vi "FieldDisp_Element_Disp.vi"(6 "Visible":bool=TRUE, 9 "Element Pose":T2 {"ROTATION"."SIN" format="%13.4f"; "ROTATION"."COS" format="%13.4f"; "ROTATION"."VALUE" format="%13.4f"; "TRANSLATION"."Y" format="%14.3f"; "TRANSLATION"."X" format="%14.3f"}, 11 "Element Info":T1) -> ()   [LabVIEW 2019, in "Trajectory_Library.lvlib"]
doc: "Displays, moves and rotates the field element on the display. \n\nInputs:\n - Element Info -- cluster -- information defining the field element.\n - Element Pose -- Pose2d -- Location and orientation of the field element.\n\nOutputs:\n -- NONE --"
uses:
  Trajectory_Library.lvlib
  TypeDef/POSE2D.ctl
  TypeDef/TRANSLATION2D.ctl
  TypeDef/ROTATION2D.ctl
  TypeDef/FieldDisp_FieldElement.ctl
  <vilib>/picture/pixmap.llb/Flatten Pixmap.vi
  <vilib>/picture/pictutil.llb/Create Mask.vi
  <vilib>/picture/picture.llb/Draw Flattened Pixmap.vi
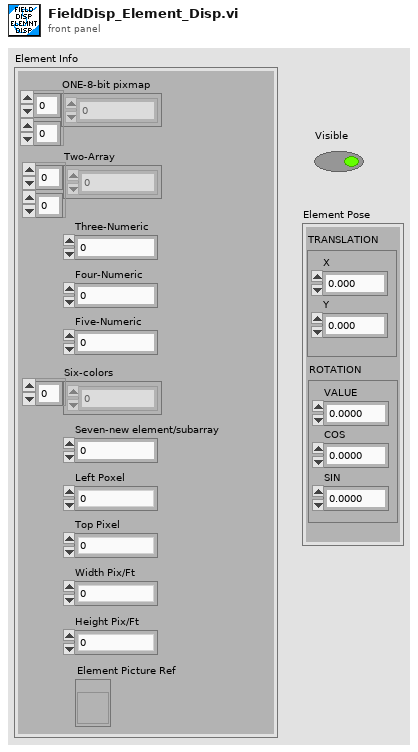
[diagram p1: front panel]
types:
  T1 = typedef "Trajectory_Library.lvlib/FieldDisp_FieldElement.ctl" = cluster{"ONE-8-bit pixmap":u8[][], "Two-Array":cdb[][], "Three-Numeric":i32, "Four-Numeric":i32, "Five-Numeric":cdb, "Six-colors":u32[], "Seven-new element/subarray":u32, "Left Poxel":dbl, "Top Pixel":dbl, "Width Pix/Ft":dbl, "Height Pix/Ft":dbl, "Element Picture Ref":refnum<vi>}
  T2 = typedef "Trajectory_Library.lvlib/POSE2D.ctl" = cluster{"TRANSLATION":T3, "ROTATION":T4}
  T3 = typedef "Trajectory_Library.lvlib/TRANSLATION2D.ctl" = cluster{"X":dbl, "Y":dbl}
  T4 = typedef "Trajectory_Library.lvlib/ROTATION2D.ctl" = cluster{"VALUE":dbl, "COS":dbl, "SIN":dbl}
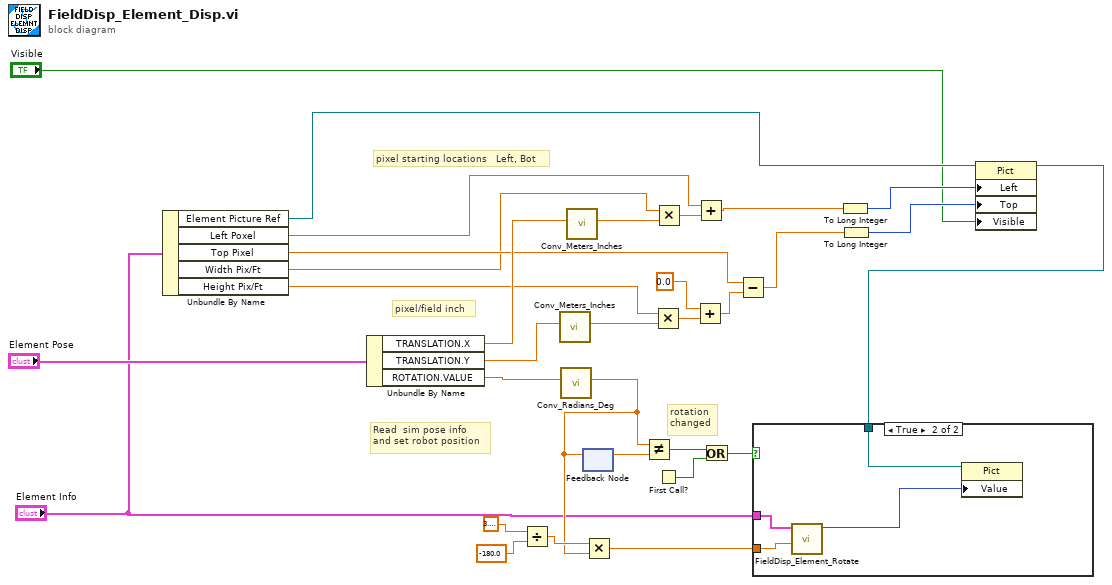
[diagram p0: block diagram]
diagram:
  # "pixel starting locations   Left, Bot"
  # "Read  sim pose info \nand set robot position"
  # "pixel/field inch"
  # "rotation\nchanged"
  n1 = Unbundle By Name("Element Info") -> ("Element Picture Ref"=w2:refnum<vi>, "Left Poxel"=w6:dbl, "Top Pixel"=w5:dbl, "Width Pix/Ft"=w4:dbl, "Height Pix/Ft"=w3:dbl)
  n2 = Unbundle By Name("Element Pose") -> ("TRANSLATION.X"=w15:dbl, "TRANSLATION.Y"=w16:dbl, "ROTATION.VALUE"=w18:dbl)
  n3 = Divide(x=3.141592653589793, y=-180.0 ("value")) -> (x/y=w27:dbl)
  n4 = call "Conv_Meters_Inches.vi"("Meters"=w16) -> ("Inches"=w22:dbl)  [unwired: 10 in]
  n5 = call "Conv_Radians_Deg.vi"("Radians"=w18) -> ("Degrees"=w17:dbl)  [unwired: 10 in]
  n6 = call "Conv_Meters_Inches.vi"("Meters"=w15) -> ("Inches"=w23:dbl)  [unwired: 10 in]
  n7 = feedback #1() -> (w8:dbl)  [unwired: 1 in]
  n8 = feedback-in #1(w17) -> ()
  n9 = Multiply(x=w27, y=w17) -> (x*y=w19:dbl)
  n10 = Not Equal?(x=w17, y=w8) -> (x != y?=w14:bool)
  n11 = Multiply(x=w3, y=w22) -> (x*y=w10:dbl)
  n12 = Multiply(x=w4, y=w23) -> (x*y=w9:dbl)
  n13 = First Call?() -> (First Call?: T/F=w28:bool)
  n14 = Add(x=0.0, y=w10) -> (x+y=w12:dbl)
  n15 = Add(x=w6, y=w9) -> (x+y=w20:dbl)
  n16 = Or(x=w14, y=w28) -> (x .or. y?=w13:bool)
  n17 = Subtract(x=w5, y=w12) -> (x-y=w21:dbl)
  n18 = To Long Integer(number=w20) -> (32bit integer=w29:i32)
  n19 = To Long Integer(number=w21) -> (32bit integer=w30:i32)
  n20 = property class="Pict"(reference=w2, "Left"=w29, "Top"=w30, "Visible"="Visible") -> (reference out=w31:refnum<vi>)  [unwired: 1 in, 1 out]
  n21 = case shown="True" w13 {
    tunnel: w19 -> [_ w34]
    tunnel: "Element Info" -> [_ w35]
    tunnel: w31 -> [_ w33]
    frame False {
    }
    frame True {
      n22 = call "FieldDisp_Element_Rotate.vi"("Angle"=w34, "RotatedPictureInfo"=w35) -> ("new picture"=w32:picture)  [unwired: 9 in]
      n23 = property class="Pict"(reference=w33, "Value"=w32) -> ()  [unwired: 1 in, 2 out]
    }
  }
